vi "staticOutputFrontEnd.vi"(8 "error in (no error)":errorcluster, 11 "StaticOutputEditor":refnum<class "StaticOutputEditor.lvclass">) -> (0 "error out":errorcluster)   [LabVIEW 2009, in "Views.lvlib" / "ScriptEditor.lvlib" / "StaticOutputEditor.lvclass"]
uses:
  StaticOutputEditor.lvclass
  StaticOutputEditor.lvclass/StaticOutputEditor.ctl
panel:
  in  "Units_Phase":string
  in  "Units_Freq":string
  in  "Phase":string
  in  "Frequency":string
  in  "Output Configuration":u16(ring) items=["", "Cooling_Light"]
  in  "Reset All":bool
  in  "Update":bool
  in  "Units":string
  in  "States":u16(ring) items=["", "cooling", "off"]
  in  "Value":string
  in  "Channel Name":u16(ring) items=["Cooling_Detuning", "analog1", "analog2", "analog3", "analog4", "analog5", "analog6", "analog7", "analogB0", "analogB1", "analogB2", "analogB3", "analogB4", "analogB5", "analogB6", "analogB7", "Pixelfly_trigger", "digital_01", "digital_02", "SpinCoreDDS0_rf_trigger", "SpinCoreDDS1_rf_trigger", "Repump_AOM", "Cooling_AOM", "Imaging_Aom", "Aom_rf3", "ethernet0", "ethernet1", "ethernet2", "ethernet3"]
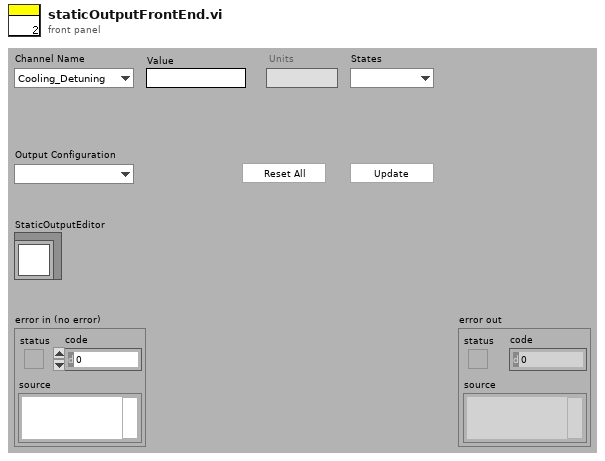
[diagram p1: front panel]
types:
  T1 = enum32{"Invalid", "Standard", "Closed", "Hidden", "Minimized", "Maximized"}
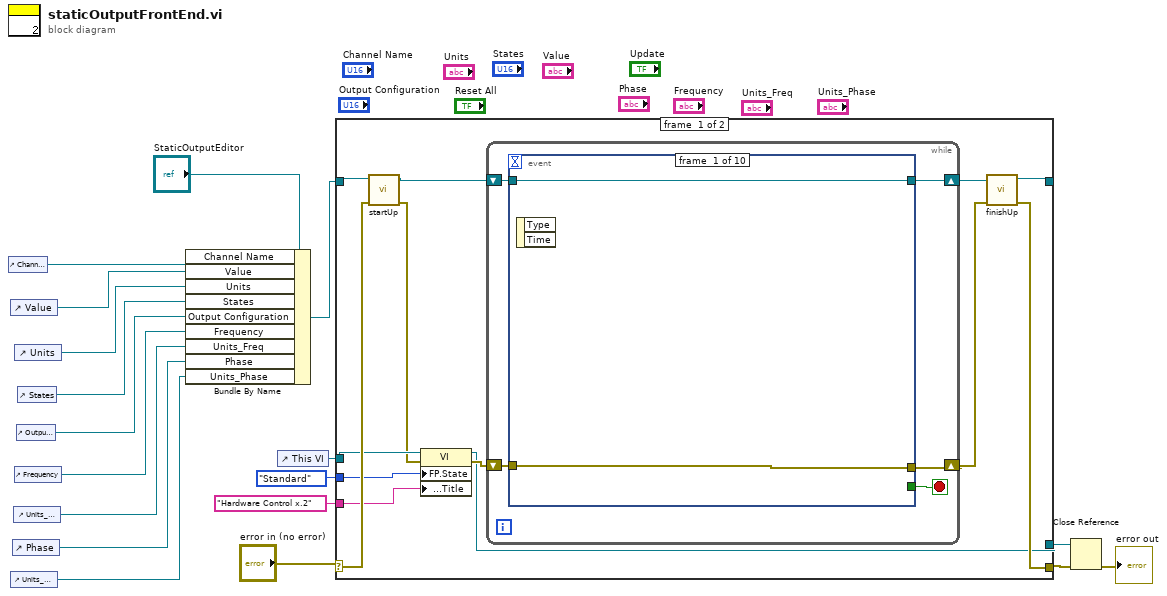
[diagram p0: block diagram]
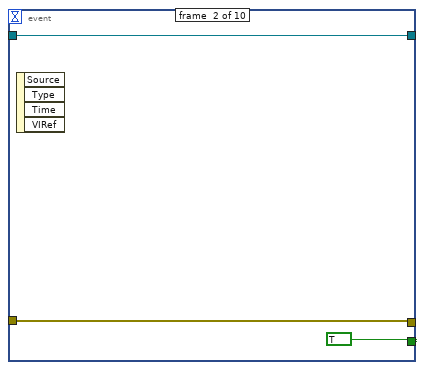
[diagram p2: hidden frame]
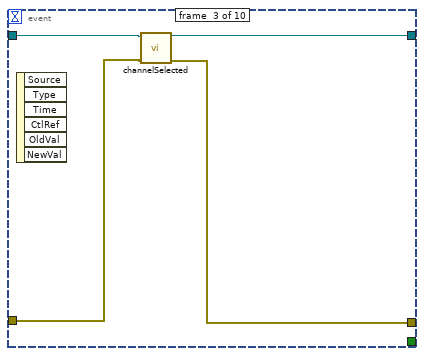
[diagram p3: hidden frame]
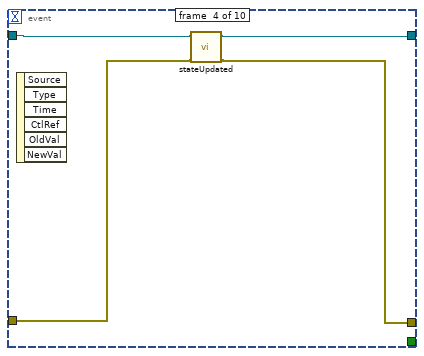
[diagram p4: hidden frame]
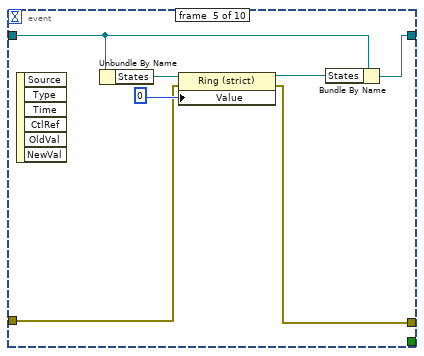
[diagram p5: hidden frame]
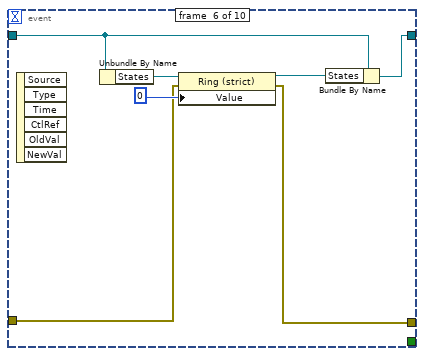
[diagram p6: hidden frame]
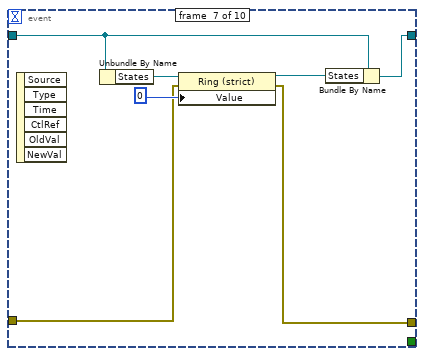
[diagram p7: hidden frame]
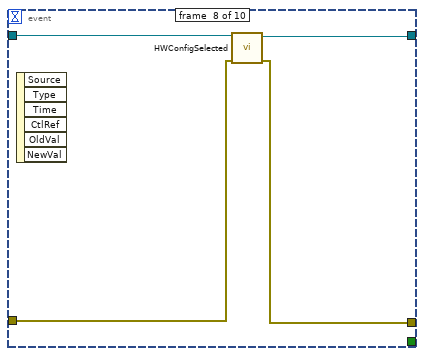
[diagram p8: hidden frame]
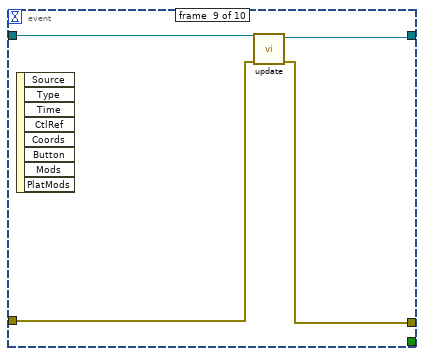
[diagram p9: hidden frame]
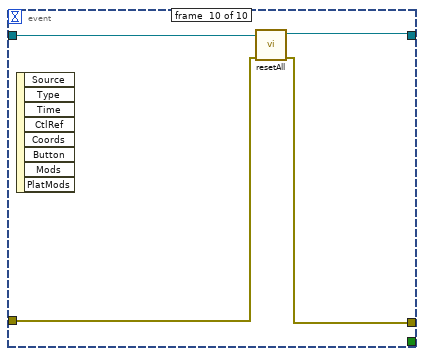
[diagram p10: hidden frame]
diagram:
  n1 = control-ref of="Channel Name"() -> (w18:refnum<vi>)
  n2 = control-ref of="Value"() -> (w17:refnum<vi>)
  n3 = control-ref of="Units_Phase"() -> (w4:refnum<vi>)
  n4 = control-ref of="Phase"() -> (w1:refnum<vi>)
  n5 = control-ref of="Units_Freq"() -> (w2:refnum<vi>)
  n6 = control-ref of="Units"() -> (w16:refnum<vi>)
  n7 = control-ref of="Frequency"() -> (w3:refnum<vi>)
  n8 = control-ref of="Output Configuration"() -> (w6:refnum<vi>)
  n9 = control-ref of="States"() -> (w15:refnum<vi>)
  n10 = Bundle By Name(cluster="StaticOutputEditor", "Channel Name"=w18, "Value"=w17, "Units"=w16, "States"=w15, "Output Configuration"=w6, "Frequency"=w3, "Units_Freq"=w2, "Phase"=w1, "Units_Phase"=w4) -> (w9:refnum<class "StaticOutputEditor.lvclass">)
  n11 = control-ref of="This VI"() -> (w13:refnum<vi>)
  n12 = case shown="No Error" "error in (no error)" {
    selector: "error in (no error)" -> [w25 w85]
    tunnel: [w28 w85] -> w11
    tunnel: [w30 w84] -> _
    tunnel: w9 -> [w27 w84]
    tunnel: w13 -> [w24 w83]
    tunnel: [w21 w83] -> w12
    tunnel: T1."Standard" ("Front Panel Window:State") -> [w20 _]
    tunnel: "Hardware Control x.2" -> [w19 _]
    frame #0 {
      n13 = call "startUp.vi"("error in (no error)"=w25, "StaticOutputEditor.lvclass"=w27) -> ("error out"=w23:errorcluster, "StaticOutputEditor.lvclass 2"=w26:refnum<class "StaticOutputEditor.lvclass">)  [unwired: 8 in]
      n14 = property class="VI"(reference=w24, error in=w23, "FP.State"=w20, "Front Panel.Title"=w19) -> (reference out=w21:refnum<vi>, error out=w22:errorcluster)
      n15 = while {
        shift-right: [w35] -> w31
        shift-left: w26 -> [w36]
        shift-right: [w34] -> w29
        shift-left: w22 -> [w32]
        stop <- w33 stop-if-true
        n16 = event shown="[1] Panel Close" {
          selector: _ -> [_ _ _ _ _ _ _ _ _ _]
          dyn-events: _ -> [_ _ _ _ _ _ _ _ _ _]
          timeout: _ -> [_ _ _ _ _ _ _ _ _ _]
          tunnel: w36 -> [w38 w39 w45 w49 w51 w58 w65 w74 w78 w82]
          tunnel: [w38 w39 w44 w48 w50 w57 w64 w73 w77 w81] -> w35
          tunnel: w32 -> [w37 w40 w43 w47 w54 w61 w68 w72 w76 w80]
          tunnel: [w37 w40 w42 w46 w53 w60 w67 w71 w75 w79] -> w34
          tunnel: [_ TRUE _ _ _ _ _ _ _ _] -> w33
          event #0 {
            n17 = event-data() -> ()  [unwired: 1 in, 2 out]
          }
          event #1 {
            n18 = event-data() -> ()  [unwired: 1 in, 4 out]
          }
          event #2 {
            n19 = event-data() -> ()  [unwired: 1 in, 6 out]
            n20 = call "channelSelected.vi"("error in (no error)"=w43, "StaticOutputEditor in"=w45) -> ("error out"=w42:errorcluster, "StaticOutputEditor out"=w44:refnum<class "StaticOutputEditor.lvclass">)  [unwired: 8 in]
          }
          event #3 {
            n21 = event-data() -> ()  [unwired: 1 in, 6 out]
            n22 = call "stateUpdated.vi"("error in (no error)"=w47, "StaticOutputEditor in"=w49) -> ("error out"=w46:errorcluster, "StaticOutputEditor out"=w48:refnum<class "StaticOutputEditor.lvclass">)  [unwired: 8 in]
          }
          event #4 {
            n23 = event-data() -> ()  [unwired: 1 in, 6 out]
            n24 = Unbundle By Name(w51) -> ("States"=w56:refnum<vi>)
            n25 = property class="Ring (strict)"(reference=w56, error in=w54, "Value"=0) -> (reference out=w52:refnum<vi>, error out=w53:errorcluster)
            n26 = Bundle By Name(cluster=w51, "States"=w52) -> (w50:refnum<class "StaticOutputEditor.lvclass">)
          }
          event #5 {
            n27 = event-data() -> ()  [unwired: 1 in, 6 out]
            n28 = Unbundle By Name(w58) -> ("States"=w63:refnum<vi>)
            n29 = property class="Ring (strict)"(reference=w63, error in=w61, "Value"=0) -> (reference out=w59:refnum<vi>, error out=w60:errorcluster)
            n30 = Bundle By Name(cluster=w58, "States"=w59) -> (w57:refnum<class "StaticOutputEditor.lvclass">)
          }
          event #6 {
            n31 = event-data() -> ()  [unwired: 1 in, 6 out]
            n32 = Unbundle By Name(w65) -> ("States"=w70:refnum<vi>)
            n33 = property class="Ring (strict)"(reference=w70, error in=w68, "Value"=0) -> (reference out=w66:refnum<vi>, error out=w67:errorcluster)
            n34 = Bundle By Name(cluster=w65, "States"=w66) -> (w64:refnum<class "StaticOutputEditor.lvclass">)
          }
          event #7 {
            n35 = event-data() -> ()  [unwired: 1 in, 6 out]
            n36 = call "HWConfigSelected.vi"("error in (no error)"=w72, "StaticOutputEditor in"=w74) -> ("error out"=w71:errorcluster, "StaticOutputEditor out"=w73:refnum<class "StaticOutputEditor.lvclass">)  [unwired: 8 in]
          }
          event #8 {
            n37 = event-data() -> ()  [unwired: 1 in, 8 out]
            n38 = call "update.vi"("error in (no error)"=w76, "StaticOutputEditor in"=w78) -> ("error out"=w75:errorcluster, "StaticOutputEditor out"=w77:refnum<class "StaticOutputEditor.lvclass">)  [unwired: 8 in]
          }
          event #9 {
            n39 = event-data() -> ()  [unwired: 1 in, 8 out]
            n40 = call "resetAll.vi"("error in (no error)"=w80, "StaticOutputEditor in"=w82) -> ("error out"=w79:errorcluster, "StaticOutputEditor out"=w81:refnum<class "StaticOutputEditor.lvclass">)  [unwired: 8 in]
          }
        }
      }
      n41 = call "finishUp.vi"("error in (no error)"=w29, "StaticOutputEditor in"=w31) -> ("error out"=w28:errorcluster, "StaticOutputEditor out"=w30:refnum<class "StaticOutputEditor.lvclass">)  [unwired: 8 in]
    }
    frame #1 {
    }
  }
  n42 = Close Reference(reference=w12, error in (no error)=w11) -> (error out=→"error out":errorcluster)
